vi "Benchmark SV Receive LV2012 - NI Verified - 1000 Byte.vi"() -> ()   [LabVIEW 2015]
panel:
  in  "1000 Byte 3":i32[][](array[numeric])
  out "1000 Byte 2":i32[][](array[numeric])
  out "1000 Byte":i32[][](array[numeric])
  in  "stop":bool
  # "Overview:  Coding that exemplifies how to benchmark the communication of Shared Variables.\nRequirements: LabVIEW 2012 or compatible\nInstructions:\n1. Run this VI\n2. Watch the amount of time it takes to communicate on the \"Benchmark SV Send  LV2012 - NI Verified.vi\" \n3. Stop both VIs"
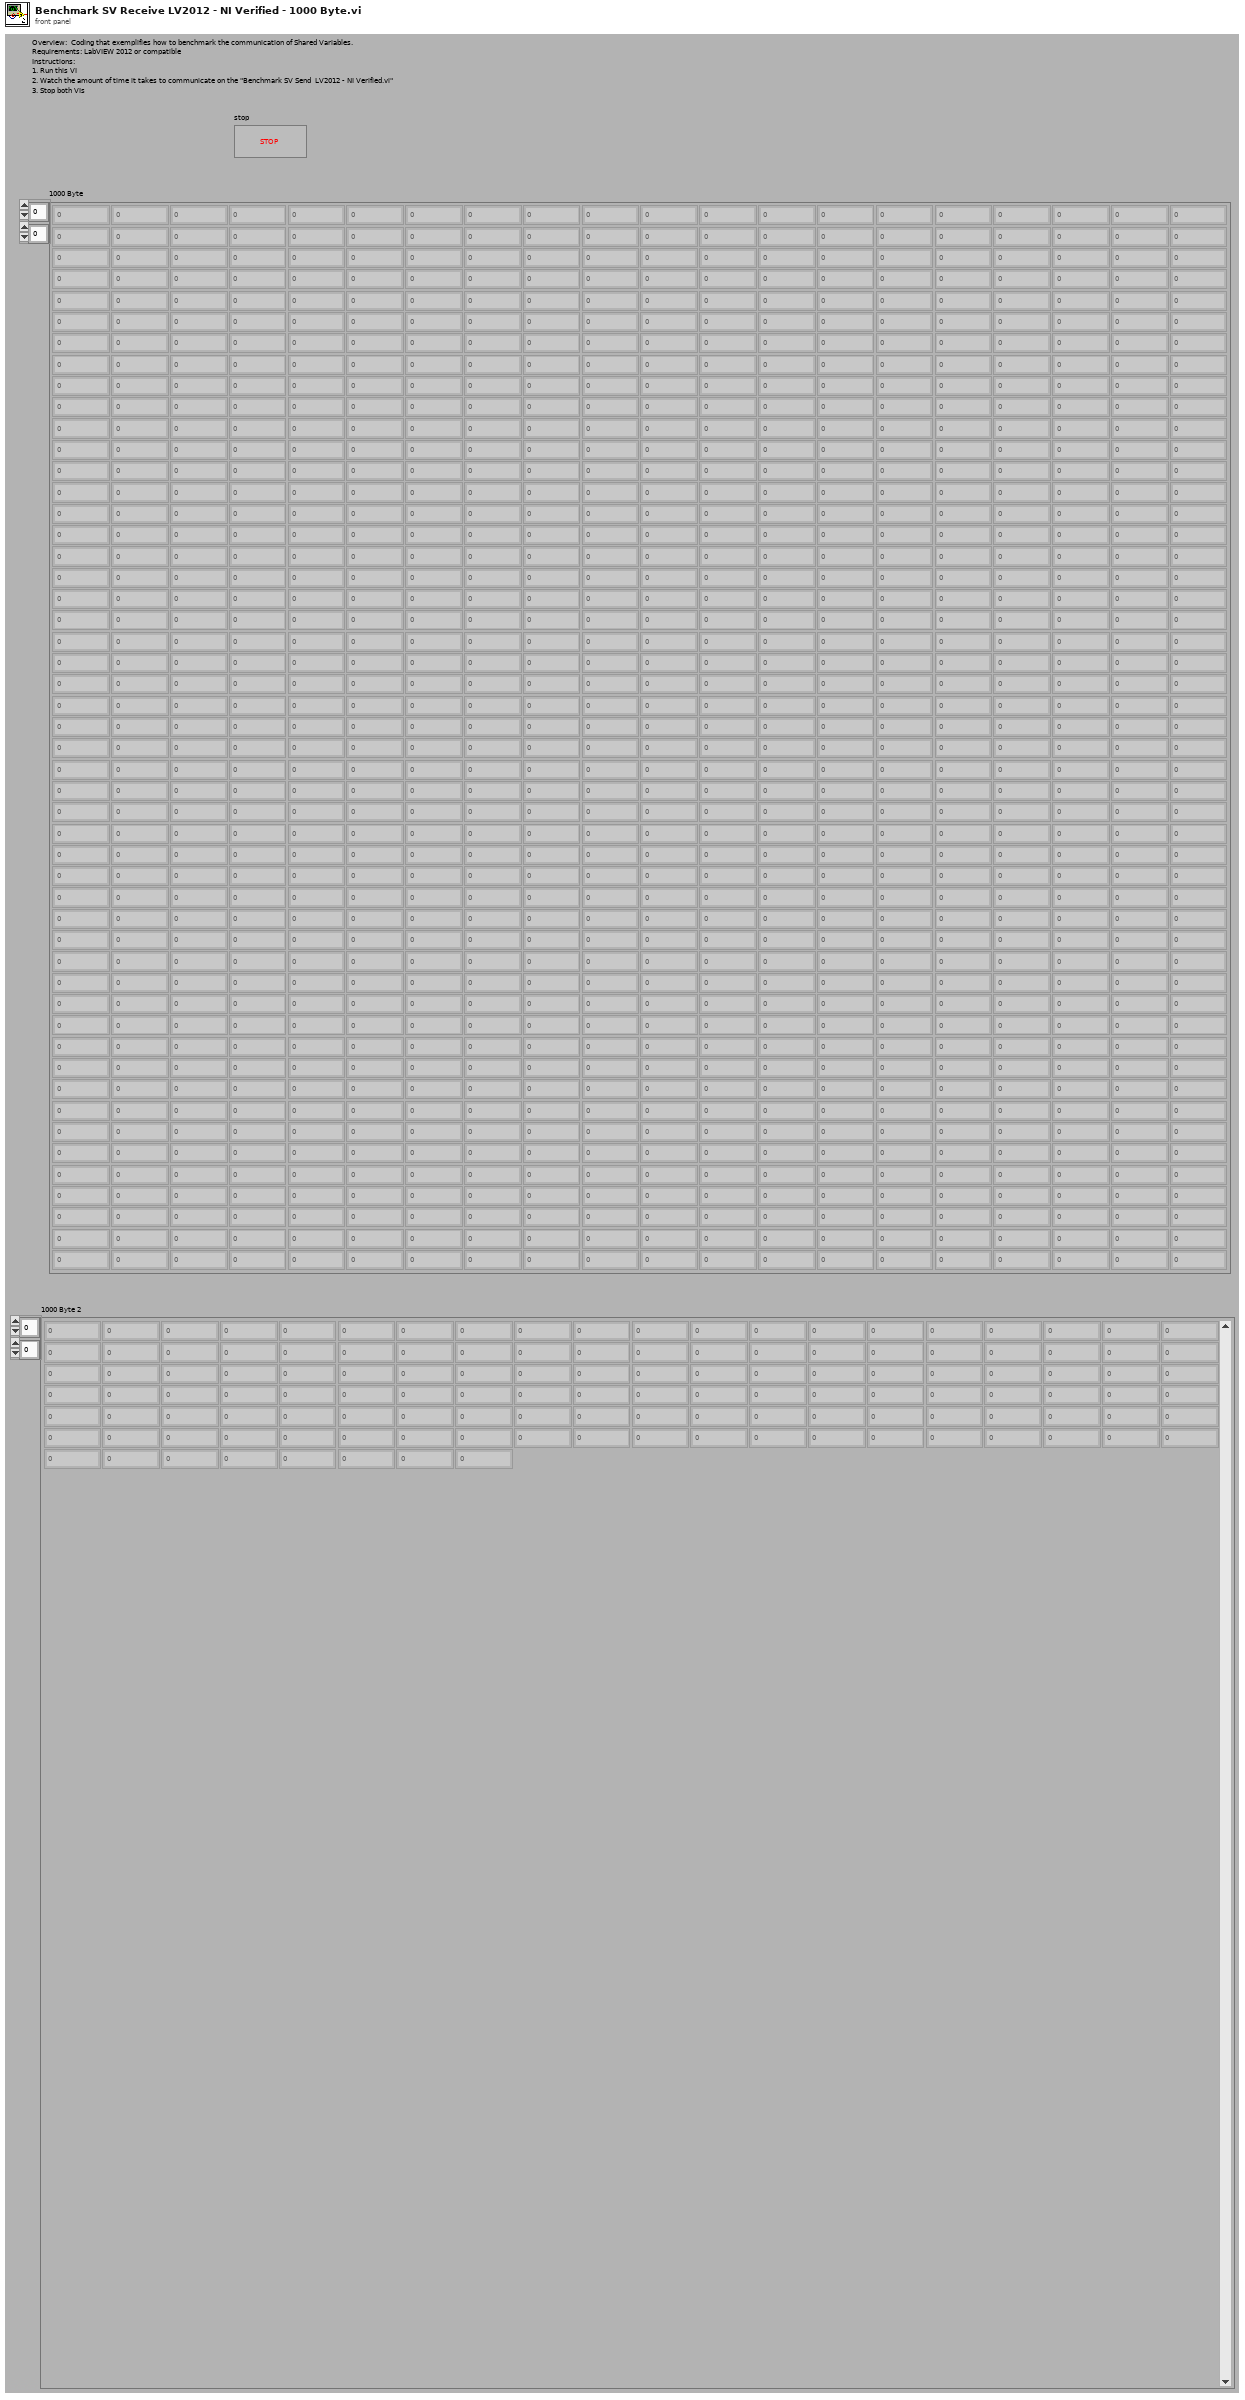
[diagram p1: front panel]
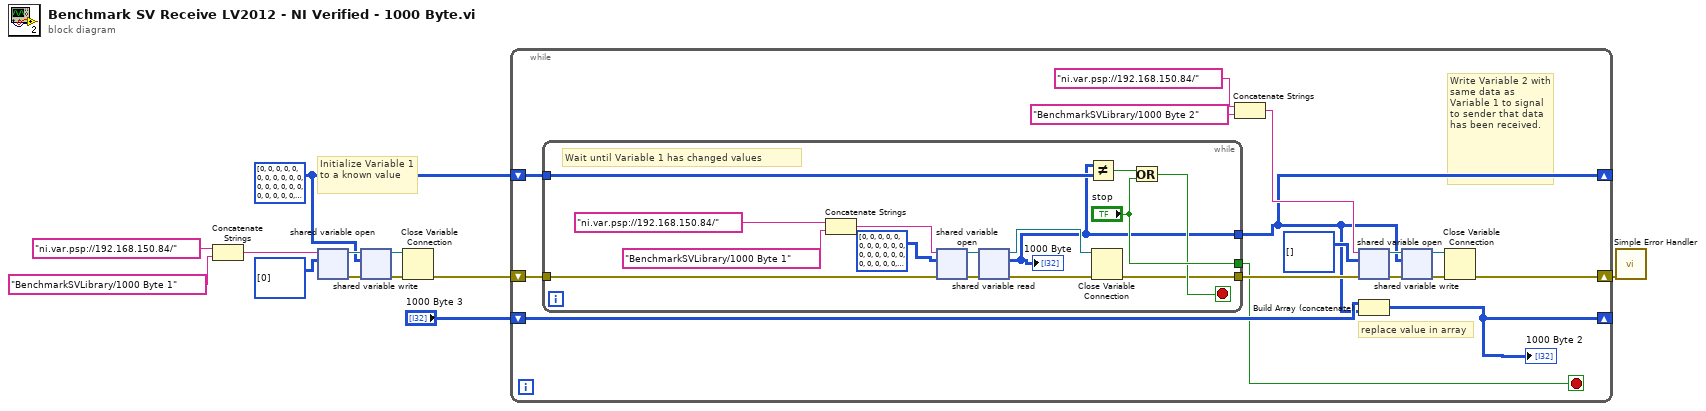
[diagram p0: block diagram]
diagram:
  w2 = i32[][] [[0, 0, 0, 0, 0, 0, 0, 0, 0, 0], [0, 0, 0, 0, 0, 0, 0, 0, 0, 0], [0, 0, 0, 0, 0, 0, 0, 0, 0, 0], [0, 0, 0, 0, 0, 0, 0, 0, 0, 0], [0, 0, 0, 0, 0, 0, 0, 0, 0, 0], [0, 0, 0, 0, 0, 0, 0, 0, 0, 0], [0, 0, 0, 0, 0, 0, 0, 0, 0, 0], [0, 0, 0, 0, 0, 0, 0, 0, 0, 0], [0, 0, 0, 0, 0, 0, 0, 0, 0, 0], [0, 0, 0, 0, 0, 0, 0, 0, 0, 0]] ("appended array")
  # "Initialize Variable 1 to a known value"
  n1 = Concatenate Strings("ni.var.psp://192.168.150.84/" ("string"), "BenchmarkSVLibrary/1000 Byte 1") -> (w11:string)
  n2 = shared-variable-open(w11, i32[][] [[0]] ("appended array")) -> (w9:refnum<k21>, w7:errorcluster)  [unwired: 2 in]
  n3 = shared-variable-write(w9, w7, w2) -> (w8:refnum<k21>, w6:errorcluster)
  n4 = Close Variable Connection(8:w6, 11:w8) -> (0:w5:errorcluster)
  n5 = while {
    shift-right: [w18] -> w12
    shift-left: w5 -> [w28]
    shift-right: [w13] -> _
    shift-left: "1000 Byte 3" -> [w16]
    shift-right: [w15] -> _
    shift-left: w2 -> [w17]
    stop <- w14 stop-if-true
    # "replace value in array"
    # "Write Variable 2 with same data as Variable 1 to signal to sender that data has been received."
    n6 = while {
      tunnel: [w29] -> w15
      tunnel: ["stop"] -> w14
      tunnel: [w35] -> w19
      tunnel: w28 -> [w34]
      tunnel: w17 -> [w31]
      stop <- w41 stop-if-true
      # "Wait until Variable 1 has changed values"
      n7 = Concatenate Strings("ni.var.psp://192.168.150.84/" ("string"), "BenchmarkSVLibrary/1000 Byte 1") -> (w32:string)
      n8 = shared-variable-open(w32, w34, i32[][] [[0, 0, 0, 0, 0, 0, 0, 0, 0, 0, 0, 0, 0, 0, 0, 0, 0, 0, 0, 0], [0, 0, 0, 0, 0, 0, 0, 0, 0, 0, 0, 0, 0, 0, 0, 0, 0, 0, 0, 0], [0, 0, 0, 0, 0, 0, 0, 0, 0, 0, 0, 0, 0, 0, 0, 0, 0, 0, 0, 0], [0, 0, 0, 0, 0, 0, 0, 0, 0, 0, 0, 0, 0, 0, 0, 0, 0, 0, 0, 0], [0, 0, 0, 0, 0, 0, 0, 0, 0, 0, 0, 0, 0, 0, 0, 0, 0, 0, 0, 0], [0, 0, 0, 0, 0, 0, 0, 0, 0, 0, 0, 0, 0, 0, 0, 0, 0, 0, 0, 0], [0, 0, 0, 0, 0, 0, 0, 0, 0, 0, 0, 0, 0, 0, 0, 0, 0, 0, 0, 0], [0, 0, 0, 0, 0, 0, 0, 0, 0, 0, 0, 0, 0, 0, 0, 0, 0, 0, 0, 0], [0, 0, 0, 0, 0, 0, 0, 0, 0, 0, 0, 0, 0, 0, 0, 0, 0, 0, 0, 0], [0, 0, 0, 0, 0, 0, 0, 0, 0, 0, 0, 0, 0, 0, 0, 0, 0, 0, 0, 0], [0, 0, 0, 0, 0, 0, 0, 0, 0, 0, 0, 0, 0, 0, 0, 0, 0, 0, 0, 0], [0, 0, 0, 0, 0, 0, 0, 0, 0, 0, 0, 0, 0, 0, 0, 0, 0, 0, 0, 0], [0, 0, 0, 0, 0, 0, 0, 0, 0, 0, 0, 0, 0, 0, 0, 0, 0, 0, 0, 0], [0, 0, 0, 0, 0, 0, 0, 0, 0, 0, 0, 0, 0, 0, 0, 0, 0, 0, 0, 0], [0, 0, 0, 0, 0, 0, 0, 0, 0, 0, 0, 0, 0, 0, 0, 0, 0, 0, 0, 0], [0, 0, 0, 0, 0, 0, 0, 0, 0, 0, 0, 0, 0, 0, 0, 0, 0, 0, 0, 0], [0, 0, 0, 0, 0, 0, 0, 0, 0, 0, 0, 0, 0, 0, 0, 0, 0, 0, 0, 0], [0, 0, 0, 0, 0, 0, 0, 0, 0, 0, 0, 0, 0, 0, 0, 0, 0, 0, 0, 0], [0, 0, 0, 0, 0, 0, 0, 0, 0, 0, 0, 0, 0, 0, 0, 0, 0, 0, 0, 0], [-1, 0, 0, 0, 0, 0, 0, 0, 0, 0, 0, 0, 0, 0, 0, 0, 0, 0, 0, 0], [0, 0, 0, 0, 0, 0, 0, 0, 0, 0, 0, 0, 0, 0, 0, 0, 0, 0, 0, 0], [0, 0, 0, 0, 0, 0, 0, 0, 0, 0, 0, 0, 0, 0, 0, 0, 0, 0, 0, 0], [0, 0, 0, 0, 0, 0, 0, 0, 0, 0, 0, 0, 0, 0, 0, 0, 0, 0, 0, 0], [0, 0, 0, 0, 0, 0, 0, 0, 0, 0, 0, 0, 0, 0, 0, 0, 0, 0, 0, 0], [0, 0, 0, 0, 0, 0, 0, 0, 0, 0, 0, 0, 0, 0, 0, 0, 0, 0, 0, 0], [0, 0, 0, 0, 0, 0, 0, 0, 0, 0, 0, 0, 0, 0, 0, 0, 0, 0, 0, 0], [0, 0, 0, 0, 0, 0, 0, 0, 0, 0, 0, 0, 0, 0, 0, 0, 0, 0, 0, 0], [0, 0, 0, 0, 0, 0, 0, 0, 0, 0, 0, 0, 0, 0, 0, 0, 0, 0, 0, 0], [0, 0, 0, 0, 0, 0, 0, 0, 0, 0, 0, 0, 0, 0, 0, 0, 0, 0, 0, 0], [0, 0, 0, 0, 0, 0, 0, 0, 0, 0, 0, 0, 0, 0, 0, 0, 0, 0, 0, 0], [0, 0, 0, 0, 0, 0, 0, 0, 0, 0, 0, 0, 0, 0, 0, 0, 0, 0, 0, 0], [0, 0, 0, 0, 0, 0, 0, 0, 0, 0, 0, 0, 0, 0, 0, 0, 0, 0, 0, 0], [0, 0, 0, 0, 0, 0, 0, 0, 0, 0, 0, 0, 0, 0, 0, 0, 0, 0, 0, 0], [0, 0, 0, 0, 0, 0, 0, 0, 0, 0, 0, 0, 0, 0, 0, 0, 0, 0, 0, 0], [0, 0, 0, 0, 0, 0, 0, 0, 0, 0, 0, 0, 0, 0, 0, 0, 0, 0, 0, 0], [0, 0, 0, 0, 0, 0, 0, 0, 0, 0, 0, 0, 0, 0, 0, 0, 0, 0, 0, 0], [0, 0, 0, 0, 0, 0, 0, 0, 0, 0, 0, 0, 0, 0, 0, 0, 0, 0, 0, 0], [0, 0, 0, 0, 0, 0, 0, 0, 0, 0, 0, 0, 0, 0, 0, 0, 0, 0, 0, 0], [0, 0, 0, 0, 0, 0, 0, 0, 0, 0, 0, 0, 0, 0, 0, 0, 0, 0, 0, 0], [0, 0, 0, 0, 0, 0, 0, 0, 0, 0, 0, 0, 0, 0, 0, 0, 0, 0, 0, 0], [0, 0, 0, 0, 0, 0, 0, 0, 0, 0, 0, 0, 0, 0, 0, 0, 0, 0, 0, 0], [0, 0, 0, 0, 0, 0, 0, 0, 0, 0, 0, 0, 0, 0, 0, 0, 0, 0, 0, 0], [0, 0, 0, 0, 0, 0, 0, 0, 0, 0, 0, 0, 0, 0, 0, 0, 0, 0, 0, 0], [0, 0, 0, 0, 0, 0, 0, 0, 0, 0, 0, 0, 0, 0, 0, 0, 0, 0, 0, 0], [0, 0, 0, 0, 0, 0, 0, 0, 0, 0, 0, 0, 0, 0, 0, 0, 0, 0, 0, 0], [0, 0, 0, 0, 0, 0, 0, 0, 0, 0, 0, 0, 0, 0, 0, 0, 0, 0, 0, 0], [0, 0, 0, 0, 0, 0, 0, 0, 0, 0, 0, 0, 0, 0, 0, 0, 0, 0, 0, 0], [0, 0, 0, 0, 0, 0, 0, 0, 0, 0, 0, 0, 0, 0, 0, 0, 0, 0, 0, 0], [0, 0, 0, 0, 0, 0, 0, 0, 0, 0, 0, 0, 0, 0, 0, 0, 0, 0, 0, 0], [0, 0, 0, 0, 0, 0, 0, 0, 0, 0, 0, 0, 0, 0, 0, 0, 0, 0, 0, 0]] ("1000 Byte")) -> (w39:refnum<k21>, w38:errorcluster)  [unwired: 1 in]
      n9 = shared-variable-read(w39, w38) -> (w37:refnum<k21>, w36:errorcluster, w29:i32[][])  [unwired: 1 out]
      "1000 Byte" <- w29
      n10 = Not Equal?(x=w29, y=w31) -> (x != y?=w43:bool)
      n11 = Close Variable Connection(8:w36, 11:w37) -> (0:w35:errorcluster)
      n12 = Or(x=w43, y="stop") -> (x .or. y?=w41:bool)
    }
    n13 = Concatenate Strings("ni.var.psp://192.168.150.84/" ("string"), "BenchmarkSVLibrary/1000 Byte 2") -> (w26:string)
    n14 = shared-variable-open(w26, w19, i32[][] [] ("appended array")) -> (w25:refnum<k21>, w24:errorcluster)  [unwired: 1 in]
    n15 = Build Array (concatenate)(w16, w15) -> (w13:i32[][])
    "1000 Byte 2" <- w13
    n16 = shared-variable-write(w25, w24, w15) -> (w23:refnum<k21>, w22:errorcluster)
    n17 = Close Variable Connection(8:w22, 11:w23) -> (0:w18:errorcluster)
  }
  n18 = call <vilib>:"Simple Error Handler.vi"("error in (no error)"=w12) -> ()  [unwired: 4 in, 5 out]
